vi "Phasor Measurement (Std 2011).vi"(0 "data in":T3, 1 "frequency configuration":T1={"channel index"=0, "nominal Fs/actual Fs"=1.0}, 2 "reset? (F)":bool, 7 "synchronization error (0.0000001 s)":dbl=1e-07 format="%#_15f", 9 "system info in":refnum<class "PMU System Info.lvclass">, 11 "error in (no error)":errorcluster, 12 "GPS information":T5[](array[typedef])) -> (3 "samples to read":u32, 4 "reporting data":T2 {"frequency" format="%#.6g"}, 6 "reporting timing information":T4 {"PMU time quality" format="%03b"; "time quality flag" format="%08b"}, 10 "system info out":refnum<class "PMU System Info.lvclass">, 14 "physical phasors":csg[](array[numeric]), 15 "error out":errorcluster)   [LabVIEW 2014, in "NI_EP_PMU.lvlib"]
doc: "Calculates the phasors, the frequency, and the rate of change of frequency at the reporting timestamp as defined in IEEE Std C37.118.1-2011."
uses:
  <vilib>/addons/Electrical Power/PMU/NI_EP_PMU.lvlib
  <vilib>/addons/Electrical Power/PMU/Common/Classes/PMU System Info/PMU System Info.lvclass
  <vilib>/addons/Electrical Power/PMU/Common/Controls/pmu_GPS Info.ctl
  <vilib>/addons/Electrical Power/PMU/Common/Controls/pmu_Reporting Time Information (Std 2011).ctl
  <vilib>/addons/Electrical Power/PMU/Common/Controls/pmu_Phasor Measurement Data.ctl
  <vilib>/addons/Electrical Power/PMU/Common/Controls/pmu_Reporting Data.ctl
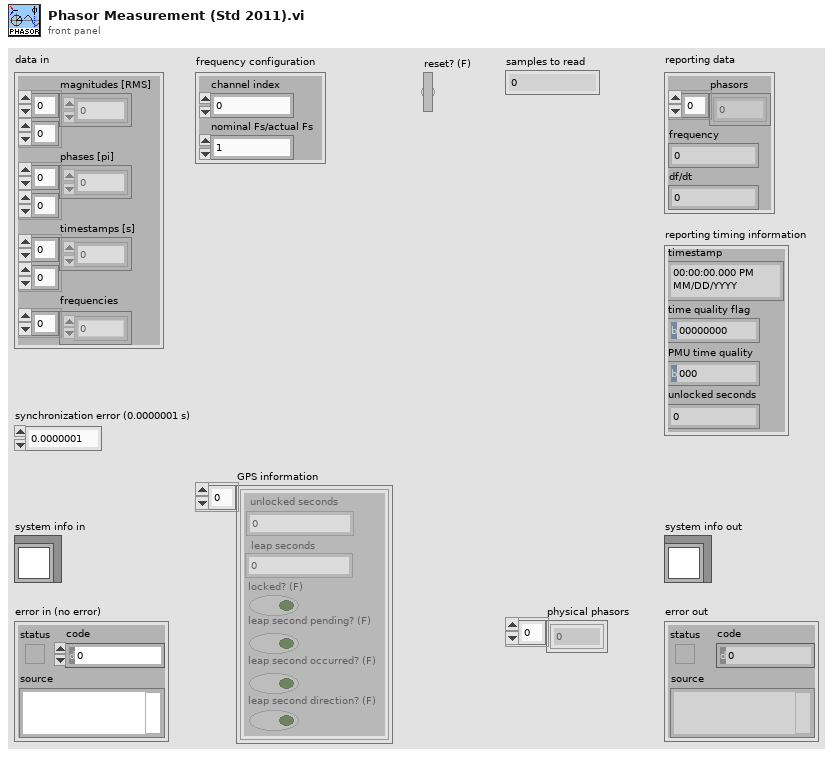
[diagram p1: front panel]
types:
  T1 = cluster{"channel index":i32, "nominal Fs/actual Fs":dbl}
  T2 = typedef "NI_EP_PMU.lvlib/pmu_Reporting Data.ctl" = cluster{"phasors":csg[], "frequency":sgl, "df/dt":sgl}
  T3 = typedef "NI_EP_PMU.lvlib/pmu_Phasor Measurement Data.ctl" = cluster{"magnitudes [RMS]":dbl[][], "phases [pi]":dbl[][], "timestamps [s]":dbl[][], "frequencies":dbl[]}
  T4 = typedef "NI_EP_PMU.lvlib/pmu_Reporting Time Information (Std 2011).ctl" = cluster{"timestamp":timestamp, "time quality flag":u8, "PMU time quality":u8, "unlocked seconds":u32}
  T5 = typedef "NI_EP_PMU.lvlib/pmu_GPS Info.ctl" = cluster{"unlocked seconds":u32, "leap seconds":i8, "locked? (F)":bool, "leap second pending? (F)":bool, "leap second occurred? (F)":bool, "leap second direction? (F)":bool}
  T6 = cluster{"reporting timestamp":dbl[], "reporting magnitudes [RMS]":dbl[], "reporting phases [pi]":dbl[]}
  T7 = cluster{"zero-crossing timestamps [s]":dbl[], "zero-crossing frequencies":dbl[]}
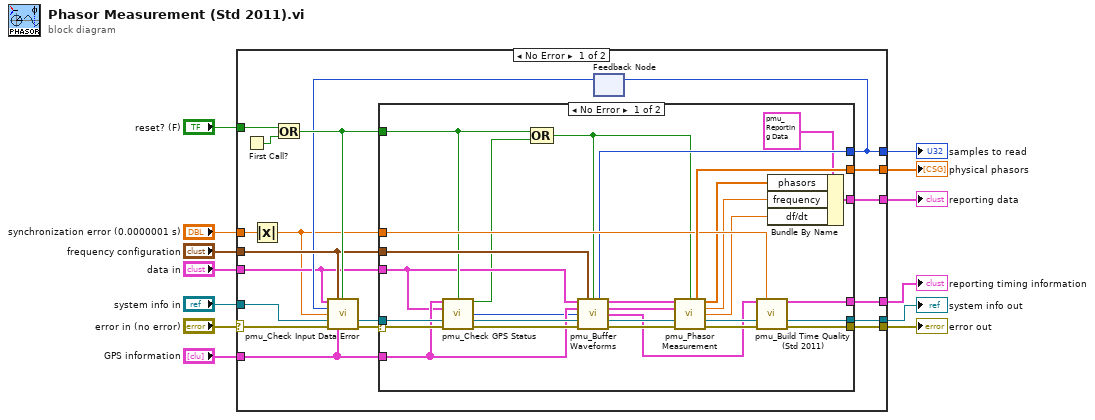
[diagram p0: block diagram]
diagram:
  n1 = case shown="No Error" "error in (no error)" {
    selector: "error in (no error)" -> [w19 w65]
    tunnel: "data in" -> [w15 _]
    tunnel: "system info in" -> [w24 w64]
    tunnel: [w32 _] -> w11
    tunnel: [w31 w64] -> w2
    tunnel: [w30 w65] -> w10
    tunnel: [w29 _] -> w9
    tunnel: "synchronization error (0.0000001 s)" -> [w25 _]
    tunnel: "frequency configuration" -> [w21 _]
    tunnel: [w17 _] -> w6
    tunnel: "GPS information" -> [w22 _]
    tunnel: "reset? (F)" -> [w27 _]
    tunnel: [w16 _] -> w1
    frame No Error {
      n2 = First Call?() -> (First Call?: T/F=w28:bool)
      n3 = Absolute Value(x=w25) -> (abs(x)=w14:dbl)
      n4 = Or(x=w27, y=w28) -> (x .or. y?=w26:bool)
      n5 = feedback #1() -> (w18:u32)  [unwired: 1 in]
      n6 = call <vilib>:"pmu_Check Input Data Error.vi"("data in"=w15, "frequency configuration"=w21, "reset? (F)"=w26, "elements need to read"=w18, "max time error [s]"=w14, "system info in"=w24, "error in (no error)"=w19, "GPS information"=w22) -> ("system info out"=w23:refnum<class "PMU System Info.lvclass">, "error out"=w20:errorcluster)  [unwired: 6 in]
      n7 = case shown="No Error" w20 {
        selector: w20 -> [w45 w63]
        tunnel: w15 -> [w34 _]
        tunnel: [w59 _] -> w32
        tunnel: [w58 w62] -> w31
        tunnel: [w57 w63] -> w30
        tunnel: [w56 _] -> w29
        tunnel: w14 -> [w53 _]
        tunnel: w21 -> [w51 _]
        tunnel: [w43 _] -> w17
        tunnel: w22 -> [w44 _]
        tunnel: w26 -> [w37 _]
        tunnel: w23 -> [w47 w62]
        tunnel: [w38 _] -> w16
        frame No Error {
          n8 = call <vilib>:"pmu_Check GPS Status.vi"("GPS information"=w44, "reset? (F)"=w37, "data in"=w34, "system info in"=w47, "error in (no error)"=w45) -> ("GPS first locking?"=w33:bool, "unlocked first index"=w35:i32, "system info out"=w48:refnum<class "PMU System Info.lvclass">, "error out"=w49:errorcluster)  [unwired: 7 in]
          n9 = Compound Arithmetic op=OR(w37, w33) -> (w36:bool)
          n10 = call <vilib>:"pmu_Buffer Waveforms.vi"("data in"=w34, "frequency configuration"=w51, "reset? (F)"=w36, "GPS information"=w44, "unlocked first index"=w35, "system info in"=w48, "error in (no error)"=w49) -> ("samples to read"=w43:u32, "reporting raw data"=w50:T6, "buffered zero-crossing frequency"=w52:T7, "reporting GPS information"=w46:T5, "system info out"=w61:refnum<class "PMU System Info.lvclass">, "error out"=w60:errorcluster)  [unwired: 3 in]
          n11 = call <vilib>:"pmu_Phasor Measurement.vi"("reporting raw data"=w50, "reset? (F)"=w36, "buffered zero-crossing frequencies"=w52, "system info in"=w61, "error in (no error)"=w60) -> ("physical phasors"=w59:csg[], "reporting phasors"=w41:csg[], "reporting frequency"=w40:sgl, "reporting df/dt"=w39:sgl, "system info out"=w55:refnum<class "PMU System Info.lvclass">, "error out"=w54:errorcluster)  [unwired: 5 in]
          n12 = call <vilib>:"pmu_Build Time Quality (Std 2011).vi"("reported GPS information"=w46, "max time error [s]"=w53, "system info in"=w55, "error in (no error)"=w54) -> ("reporting timing information"=w56:T4, "system info out"=w58:refnum<class "PMU System Info.lvclass">, "error out"=w57:errorcluster)  [unwired: 9 in]
          n13 = Bundle By Name(cluster=T2 {"phasors"=[0.011429072-99.96636i, -86.60898+49.966427i, 86.59466+50.004635i, 0.00039273032-0.9994094i, 0.00039950816-0.9995112i, 0.00037330666-0.9995143i], "frequency"=49.999996, "df/dt"=0.00031614315} ("reporting data"), "phasors"=w41, "frequency"=w40, "df/dt"=w39) -> (w38:T2)
        }
        frame Error {
        }
      }
      n14 = feedback-in #1(w17) -> ()
    }
    frame Error {
    }
  }
  "error out" <- w10
  "system info out" <- w2
  "reporting timing information" <- w9
  "reporting data" <- w1
  "physical phasors" <- w11
  "samples to read" <- w6
